vi "Update Icon Preview.vi"(7 "Icon Text":string, 8 "error in (no error)":errorcluster, 9 "Instrument  Color":u32, 10 "Instrument Text Color":u32, 11 "Icon.lvclass in":refnum<class "Icon.lvclass">) -> (0 "error out":errorcluster, 2 "new picture":picture, 3 "lv_icon.lvlib:Icon.lvclass out":refnum<class "Icon.lvclass">)   [LabVIEW 2019, in "ProjectItem.lvclass"]
uses:
  ProjectItem.lvclass
  <vilib>/LabVIEW Icon API/lv_icon/Classes/Icon/Icon.lvclass
  <vilib>/LabVIEW Icon API/API_Rectangle Dimension.ctl
  <vilib>/LabVIEW Icon API/API_Text.ctl
  <vilib>/LabVIEW Icon API/API_Rectangle Colors.ctl
  <vilib>/LabVIEW Icon API/API_Test Settings.ctl
  <vilib>/LabVIEW Icon API/lv_icon/Controls/Alignment.ctl
  <vilib>/LabVIEW Icon API/API_Text Colors.ctl
  <vilib>/LabVIEW Icon API/LabVIEW Icon API.lvlib
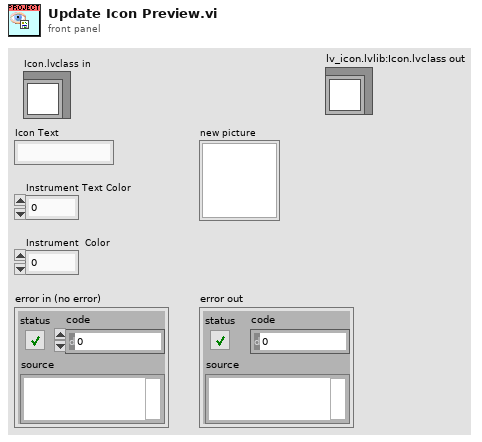
[diagram p1: front panel]
types:
  T1 = typedef "LabVIEW Icon API.lvlib/API_Test Settings.ctl" = cluster{"Font":string, "Alignment":T2, "Size":u8, "Center text":bool, "Capitalize text":bool, "Text color":T3}
  T2 = typedef "Alignment.ctl" = u16
  T3 = typedef "LabVIEW Icon API.lvlib/API_Text Colors.ctl" = cluster{"Line 1 color":u32, "Line 2 color":u32, "Line 3 color":u32, "Line 4 color":u32}
  T4 = typedef "LabVIEW Icon API.lvlib/API_Rectangle Colors.ctl" = cluster{"Border":u32, "Background":u32}
  T5 = typedef "LabVIEW Icon API.lvlib/API_Text.ctl" = cluster{"Line 1 text":string, "Line 2 text":string, "Line 3 text":string, "Line 4 text":string}
  T6 = typedef "LabVIEW Icon API.lvlib/API_Rectangle Dimension.ctl" = cluster{"Width":i16, "Height":i16}
  T7 = typedef "imagedata.ctl" = cluster{"image type":i32, "image depth":i32, "image":u8[], "mask":u8[], "colors":u32[], "Rectangle":cluster{"left":i16, "top":i16, "right":i16, "bottom":i16}}
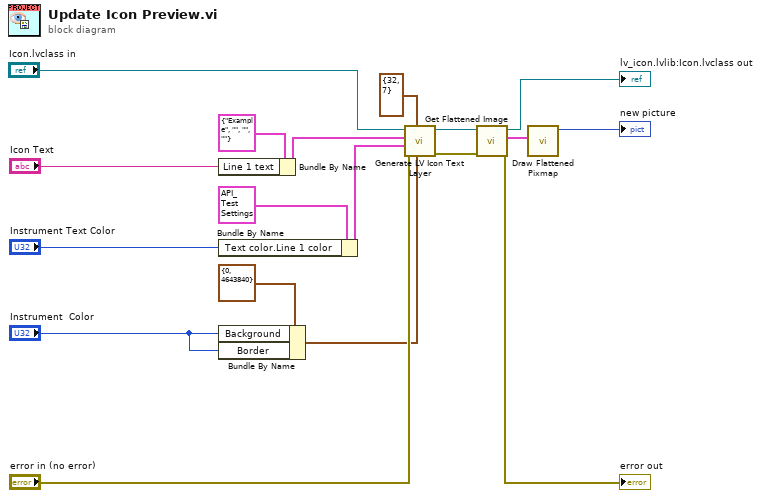
[diagram p0: block diagram]
diagram:
  n1 = Bundle By Name(cluster=T5 {"Line 1 text"="Example", "Line 2 text"="", "Line 3 text"="", "Line 4 text"=""} ("Text"), "Line 1 text"="Icon Text") -> (w13:T5)
  n2 = Bundle By Name(cluster=T1 {"Font"="Small Fonts", "Alignment"=1, "Size"=8, "Center text"=TRUE, "Capitalize text"=TRUE, "Text color"={"Line 1 color"=0, "Line 2 color"=0, "Line 3 color"=0, "Line 4 color"=0}} ("Text settings"), "Text color.Line 1 color"="Instrument Text Color") -> (w11:T1)
  n3 = Bundle By Name(cluster=T4 {"Border"=0, "Background"=4643840} ("Rectangle colors (black, white)"), "Background"="Instrument  Color", "Border"="Instrument  Color") -> (w10:T4)
  n4 = call <vilib>:"Generate LV Icon Text Layer.vi"("Rectangle colors (black, white)"=w10, "Rectangle dimension (32,32)"=T6 {"Width"=32, "Height"=7}, "error in (no error)"="error in (no error)", "Text settings"=w11, "Text"=w13, "Icon in"="Icon.lvclass in") -> ("error out"=w16:errorcluster, "Icon out"=w8:refnum<class "Icon.lvclass">)  [unwired: 4 in]
  n5 = call <vilib>:"Get Flattened Image.vi"("error in (no error)"=w16, "lv_icon.lvlib:Icon.lvclass in"=w8) -> ("error out"=→"error out":errorcluster, "Color Image"=w7:T7, "lv_icon.lvlib:Icon.lvclass out"=→"lv_icon.lvlib:Icon.lvclass out":refnum<class "Icon.lvclass">)  [unwired: 6 in, 1 out]
  n6 = call <vilib>:"Draw Flattened Pixmap.vi"("image data"=w7) -> ("new picture"=→"new picture":picture)  [unwired: 8 in]
